vi "LastLine.vi"(11 "Reply":string) -> (3 "String":string)   [LabVIEW 2019]
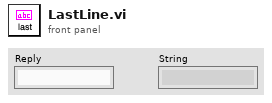
[diagram p1: front panel]
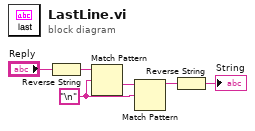
[diagram p0: block diagram]
diagram:
  w4 = "\n" ("regular expression")
  n1 = Reverse String(1:"Reply") -> (0:w2:string)
  n2 = Match Pattern(string=w2, regular expression=w4) -> (after substring=w3:string)  [unwired: 1 in, 3 out]
  n3 = Match Pattern(string=w3, regular expression=w4) -> (before substring=w5:string)  [unwired: 1 in, 3 out]
  n4 = Reverse String(1:w5) -> (0:→"String":string)
